vi "EnqueError.vi"(11 "ErrorArrayIn":errorcluster[](array[cluster])) -> (3 "ErrorArrayOut":errorcluster[](array[cluster]))   [LabVIEW 2018, in "Queue.lvlib"]
uses:
  Queue.lvlib
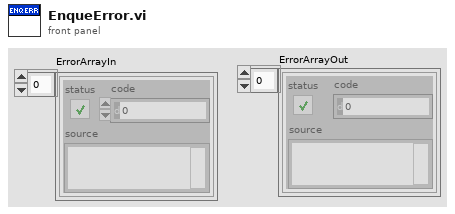
[diagram p1: front panel]
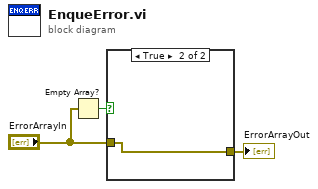
[diagram p0: block diagram]
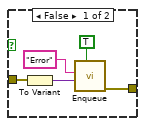
[diagram p2: hidden frame]
diagram:
  n1 = Empty Array?(array="ErrorArrayIn") -> (empty?=w3:bool)
  n2 = case shown="True" w3 {
    tunnel: "ErrorArrayIn" -> [w7 w9]
    tunnel: [w4 w9] -> w1
    frame False {
      n3 = To Variant(anything=w7) -> (Variant=w8:variant)
      n4 = call "Enqueue.vi"("Priority (F)"=TRUE, "Message Data"=w8, "Message"="Error") -> ("ErrorArray"=w4:errorcluster[])  [unwired: 8 in]
    }
    frame True {
    }
  }
  "ErrorArrayOut" <- w1
